vi "Destroy.vi"(0 "reference in":refnum<class "IQBurst_memo.lvclass">, 5 "error in (no error)":errorcluster) -> (14 "reference out":refnum<class "IQBurst_memo.lvclass">, 19 "error out":errorcluster)   [LabVIEW 2019, in "IQBurst_memo.lvclass"]
doc: "Destructor."
uses:
  IQBurst_memo.lvclass
  mmWave data_class/mmWave data.lvclass
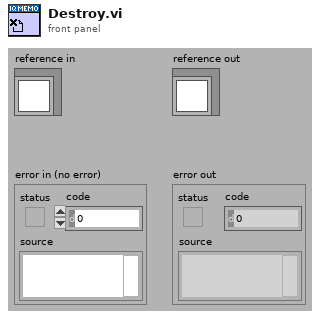
[diagram p1: front panel]
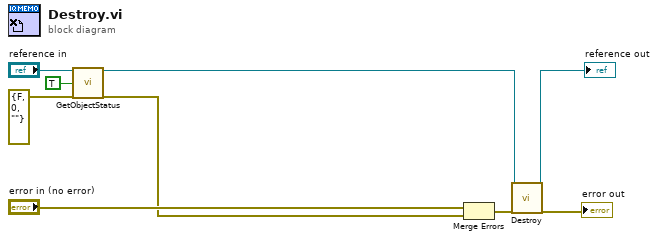
[diagram p0: block diagram]
diagram:
  n1 = call-dynamic "GetObjectStatus.vi"("reference in"="reference in", "simple info (F)"=TRUE ("simple info"), "error in (no error)"=errorcluster {"status"=FALSE, "code"=0, "source"=""}) -> ("reference out"=w1:refnum<class "IQBurst_memo.lvclass">, "error out"=w2:errorcluster)  [unwired: 5 in, 10 out]
  n2 = Merge Errors("error in (no error)", w2) -> (w8:errorcluster)
  n3 = call-parent "Destroy.vi"("reference in"=w1, "error in (no error)"=w8) -> ("reference out"=→"reference out":refnum<class "IQBurst_memo.lvclass">, "error out"=→"error out":errorcluster)  [unwired: 16 in]
